vi "NI VeriStand - Set Multiple Parameter 2D Array Values.vi"(7 "Target":string, 8 "error in (no error)":errorcluster, 9 "Data Array":T1[](array[typedef]), 10 "Parameters":string[](array[string]), 11 "ModelManager in":T2) -> (0 "error out":errorcluster, 3 "ModelManager out":T2)   [LabVIEW 2020, in "NI_VS ModelManager ExecutionAPI.lvlib"]
doc: "Sets values of model parameters present on the target. You must manually select the polymorphic instance to use."
uses:
  <vilib>/NI VeriStand/Execution/ModelManager/NI_VS ModelManager ExecutionAPI.lvlib
  <vilib>/NI VeriStand/Execution/ModelManager/ModelManagerAPI.ctl
  NationalInstruments.VeriStand.ClientAPI
  <vilib>/NI VeriStand/Execution/ModelManager/2D Array of Double.ctl
  NationalInstruments.VeriStand
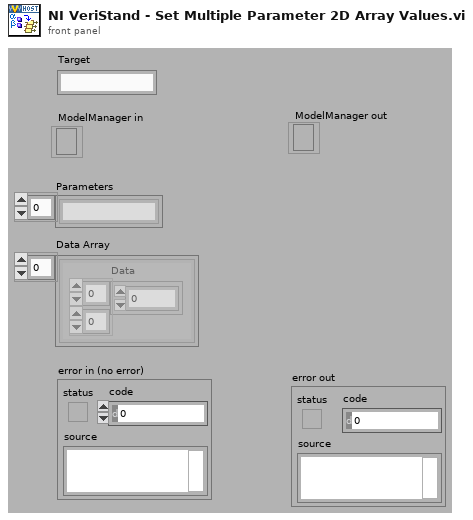
[diagram p1: front panel]
types:
  T1 = typedef "NI_VS ModelManager ExecutionAPI.lvlib/2D Array of Double.ctl" = cluster{"Data":dbl[][]}
  T2 = typedef "NI_VS ModelManager ExecutionAPI.lvlib/ModelManagerAPI.ctl" = refnum<k24>
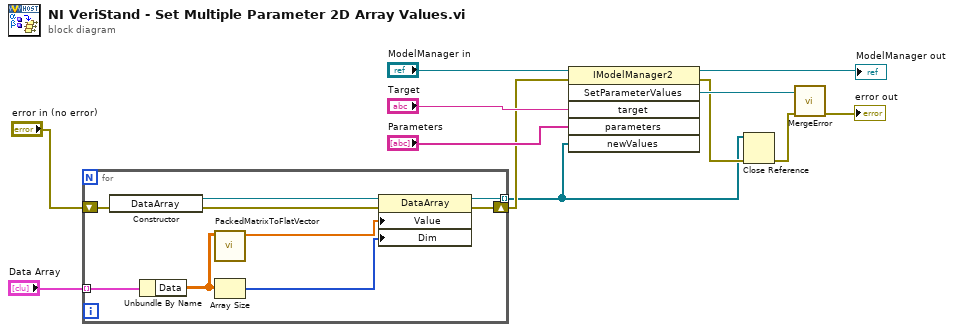
[diagram p0: block diagram]
diagram:
  n1 = for {
    tunnel: [w20] -> w1 mode=indexing
    tunnel: "Data Array" -> [w19] mode=indexing
    shift-right: [w13] -> w4
    shift-left: "error in (no error)" -> [w14]
    n2 = constructor class="DataArray"(error in=w14) -> (reference out=w21:refnum<k24>, error out=w15:errorcluster)  [unwired: 2 in, 1 out]
    n3 = Unbundle By Name(w19) -> ("Data"=w17:dbl[][])
    n4 = call <vilib>:"PackedMatrixToFlatVector.vi"("Matrix"=w17) -> ("FlatVector"=w16:dbl[])  [unwired: 10 in]
    n5 = Array Size(array=w17) -> (size(s)=w18:i32[])
    n6 = property class="DataArray"(reference=w21, error in=w15, "Value"=w16, "Dim"=w18) -> (reference out=w20:refnum<k24>, error out=w13:errorcluster)
  }
  n7 = invoke class="IModelManager2" method="SetParameterValues"(reference="ModelManager in", error in=w4, "target"="Target", "parameters"="Parameters", "newValues"=w1) -> (reference out=→"ModelManager out":T2, error out=w3:errorcluster, "SetParameterValues"=w12:refnum<k24>)  [unwired: 1 in, 3 out]
  n8 = Close Reference(reference=w1, error in (no error)=w3) -> (error out=w2:errorcluster)
  n9 = call <vilib>:"MergeError.vi"("error in (no error)"=w2, "Error"=w12) -> ("error out"=→"error out":errorcluster)  [unwired: 9 out]
